vi "coerce_command.vi"(1 "U8 code":u8) -> (0 "Command":T1)   [LabVIEW 2012]
uses:
  Common/i2c_command.ctl
panel:
  # "Coerce a U8 into an \"I2C command\" enum."
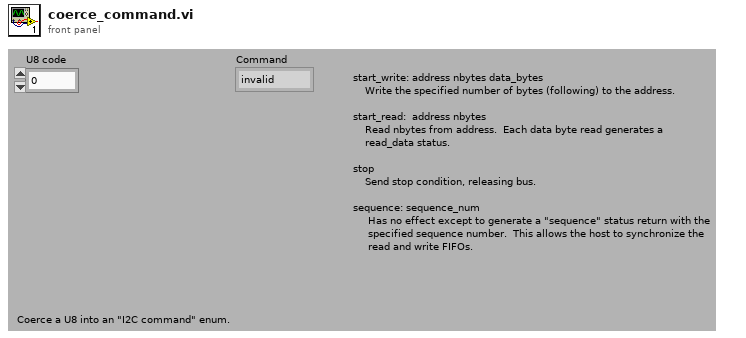
[diagram p1: front panel]
types:
  T1 = typedef "i2c_command.ctl" = enum8{"invalid", "start_write", "start_read", "stop", "sequence"}
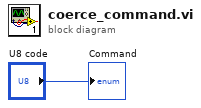
[diagram p0: block diagram]
diagram:
  "Command" <- "U8 code"
